vi "Get Cam Focus.vi"() -> ()   [LabVIEW 2015]
uses:
  <vilib>/Utility/file.llb/Read Delimited Spreadsheet (string).vi
  <vilib>/Utility/file.llb/Write Delimited Spreadsheet (string).vi
  Users/Stephen/Desktop/BETA_GSCS - Copy/Systems/SIcamera_Control/SIcamera_Globals.vi
panel:
  in  "Array":string[][](array[string])
  in  "Save":bool
  in  "Line Number":dbl=1.0
  in  "Open script":bool
  in  "Current Script":string[][](table)
  in  "text file":refnum<file>
  in  "Script Name":string
  out "status":string
  in  "Add to Script Button":bool
  in  "Location of Script File":path=path "C:/GSCS Scripting/Scripts"
  in  "cluster":T1={"Path to Configuration File"=path "", "SI camera info"={"Exp time"=0.0, "Number of Exp"=0.0, "Exp type tab"=enum."Object", "CCD ROI Mode"=10, "File name base"="", "Camera Color"="Red", "Notes"="", "Observer Name"="", "object name"="", "CCD Readout Speed"=5, "Hg(Ar)"=FALSE, "Cu"=FALSE, "Ne"=FALSE, "Ar"=FALSE, "Quartz"=FALSE, "Fe"=FALSE, "Bulb"=FALSE, "Quartz Percent"=0.0, "Cam Focus"=0.0}} {"SI camera info"."CCD Readout Speed" items=["750 kHz, ATTN 0", "750 kHz, ATTN 2", "344 kHz, ATTN 0", "344 kHz, ATTN 3", "100 kHz, ATTN 2", "100 kHz, ATTN 3"]; "SI camera info"."CCD ROI Mode" items=["Imaging, 1x1  "=0, "Imaging, 2x2"=1, "Imaging, 3x3"=2, "Spectroscopic, 1x1"=3, "Spectroscopic, 2x2"=4, "Spectroscopic, 3x3"=5, "MOS, 1x1"=11, "MOS, 2x2"=12, "MOS, 3x3"=13, "Slicer"=6, "Spectroscopic, ZZ Ceti"=14, "Slit Imaging/Alignment"=7, "MOS Imaging/Alignment"=10, "Set user-defined ROI..."=21, "Custom Mode"=9]}
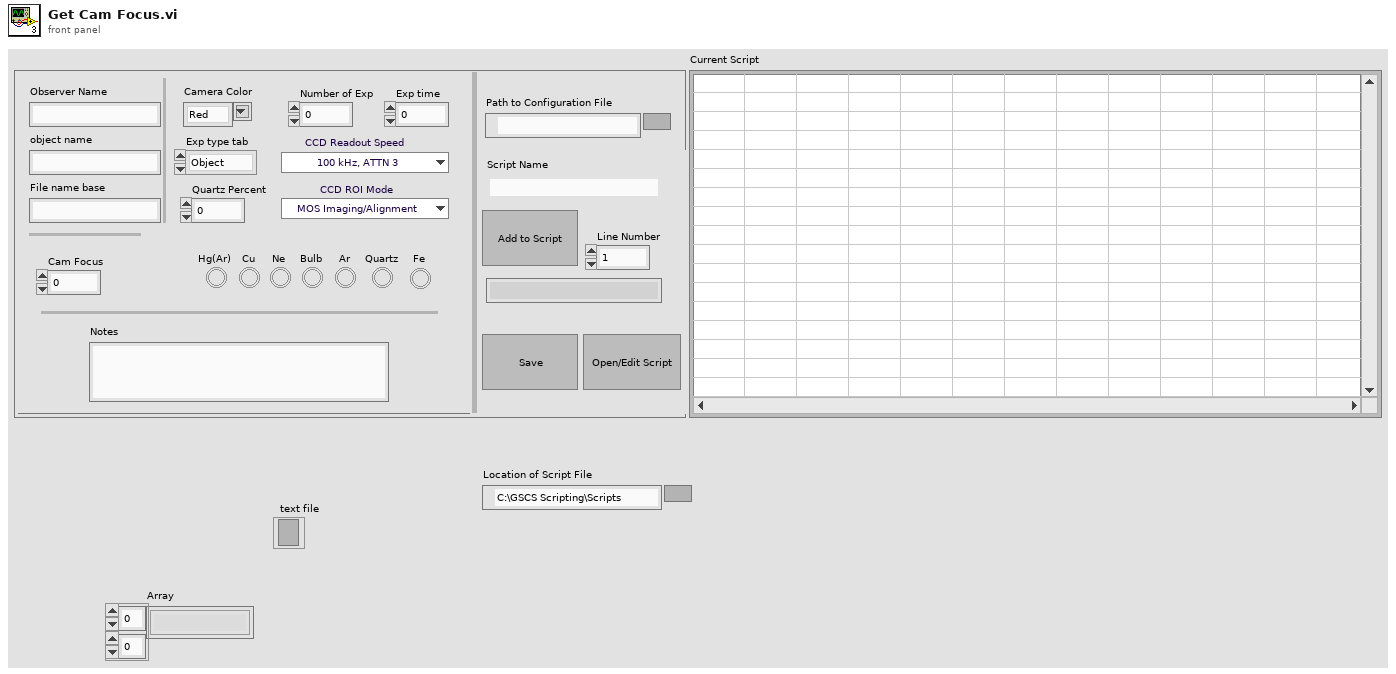
[diagram p1: front panel]
types:
  T1 = cluster{"Path to Configuration File":path, "SI camera info":cluster{"Exp time":dbl, "Number of Exp":dbl, "Exp type tab":enum16{"Object", "Flat", "Comp", "Dark", "Zero"}, "CCD ROI Mode":u16, "File name base":string, "Camera Color":string, "Notes":string, "Observer Name":string, "object name":string, "CCD Readout Speed":u8, "Hg(Ar)":bool, "Cu":bool, "Ne":bool, "Ar":bool, "Quartz":bool, "Fe":bool, "Bulb":bool, "Quartz Percent":dbl, "Cam Focus":dbl}}
  T2 = cluster{"Serial Origin":i32, "Serial Length":i32, "Serial Binning":i32, "Parallel Origin":i32, "Parallel Length":i32, "Parallel Binning":i32}
  T3 = typedef "LVPoint32TypeDef.ctl" = cluster{"Horizontal":i32, "Vertical":i32}
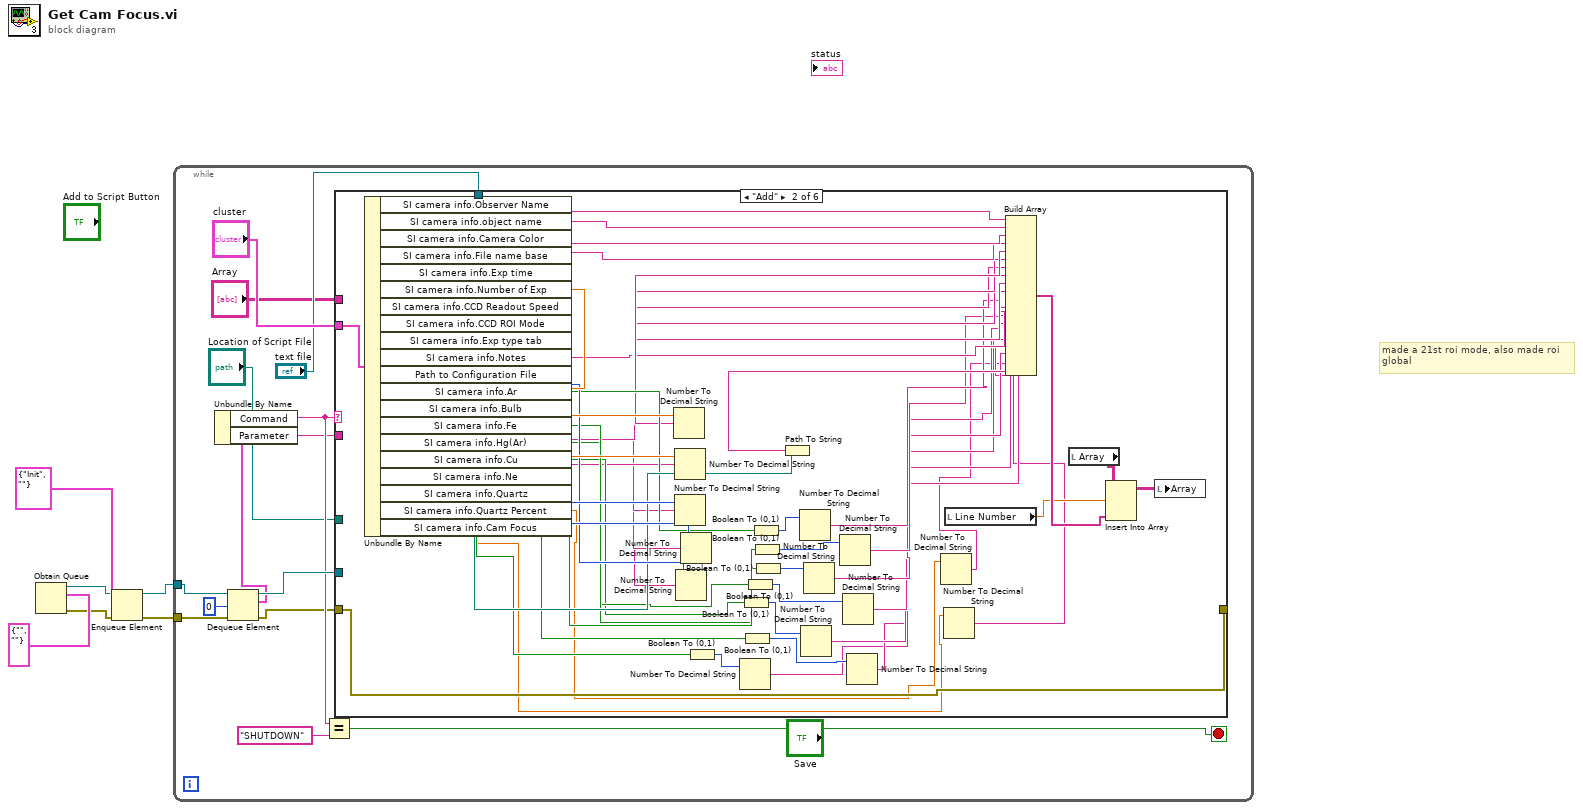
[diagram p0: block diagram]
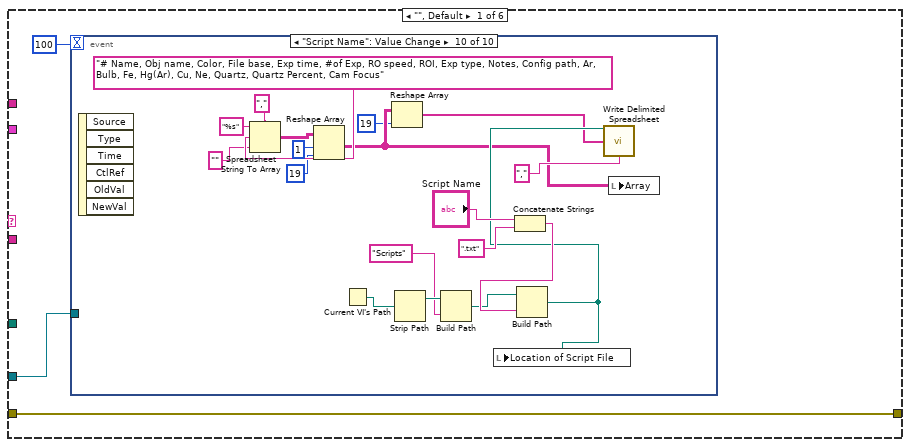
[diagram p2: hidden frame]
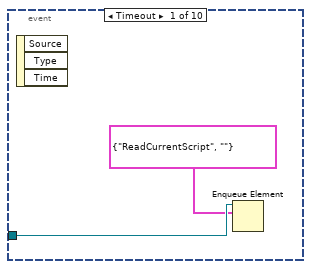
[diagram p3: hidden frame]
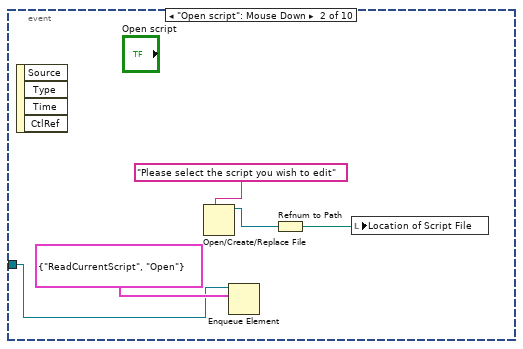
[diagram p4: hidden frame]
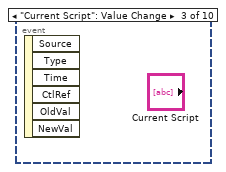
[diagram p5: hidden frame]
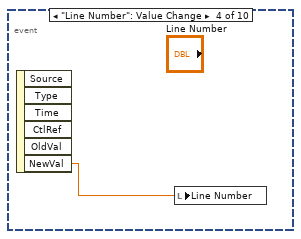
[diagram p6: hidden frame]
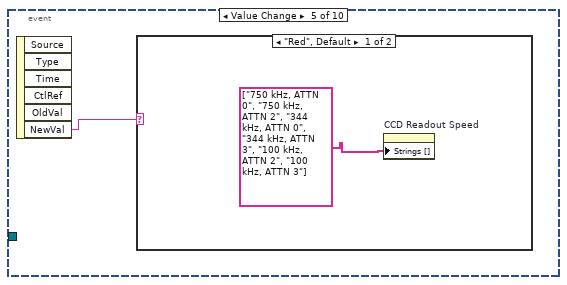
[diagram p7: hidden frame]
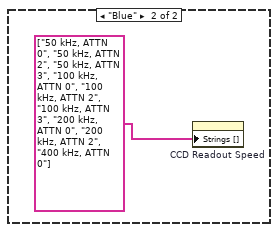
[diagram p8: hidden frame]
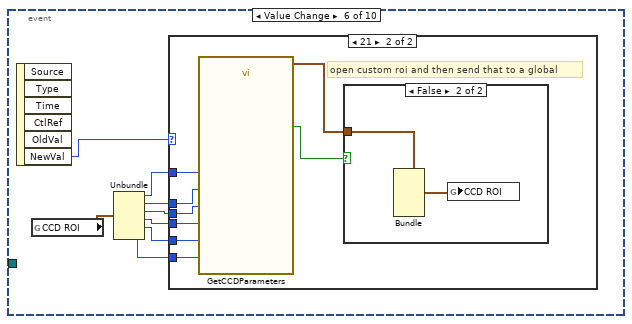
[diagram p9: hidden frame]
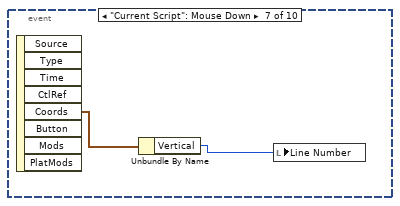
[diagram p12: hidden frame]
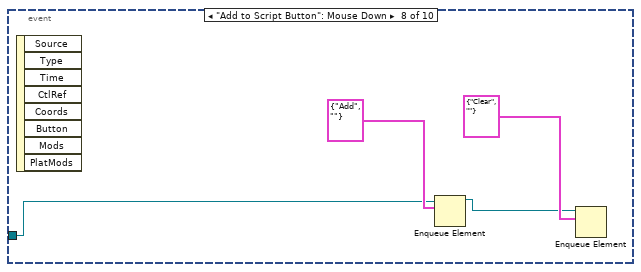
[diagram p13: hidden frame]
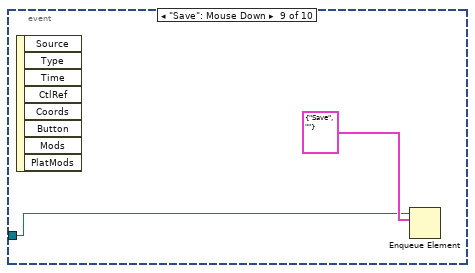
[diagram p14: hidden frame]
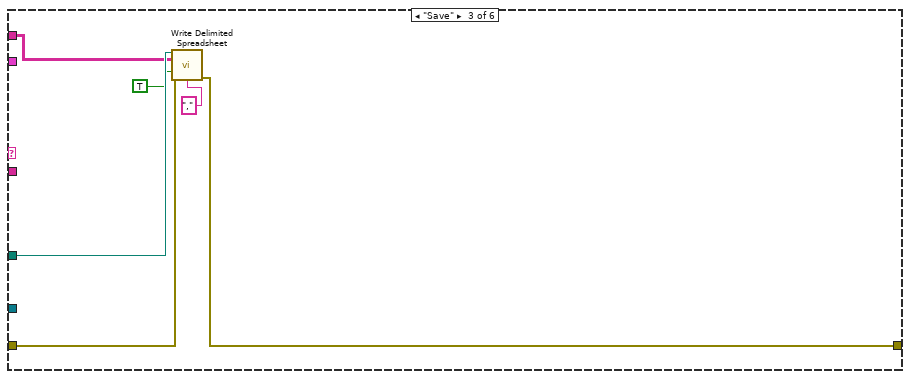
[diagram p15: hidden frame]
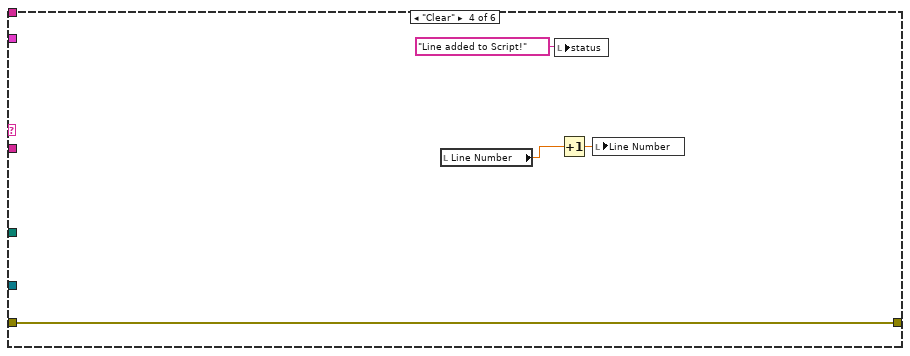
[diagram p16: hidden frame]
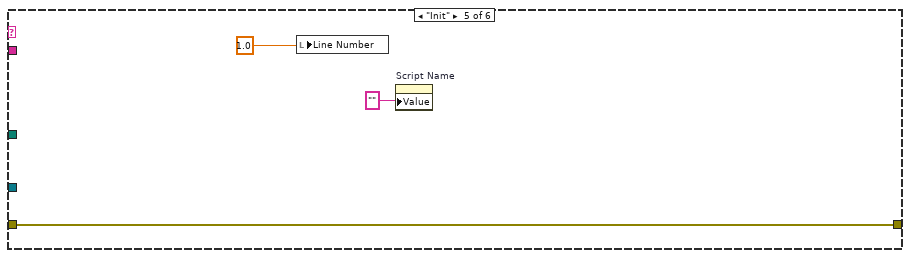
[diagram p17: hidden frame]
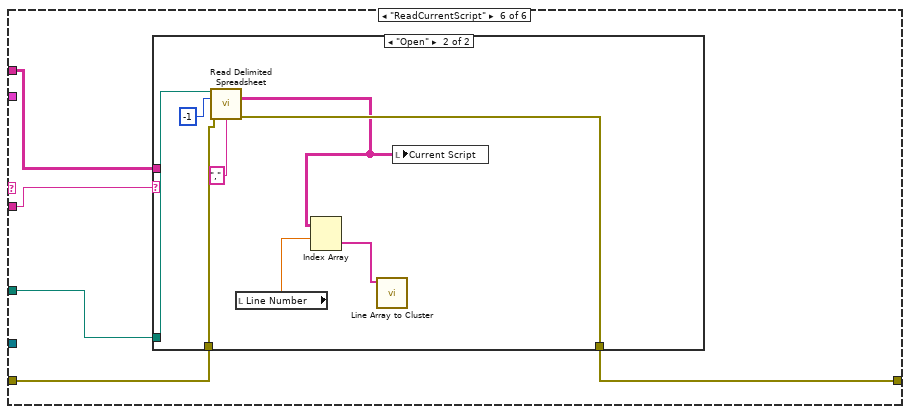
[diagram p18: hidden frame]
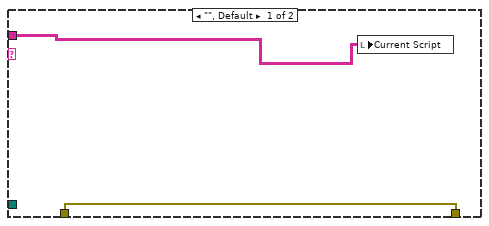
[diagram p19: hidden frame]
diagram:
  # "made a 21st roi mode, also made roi\nglobal"
  n1 = Obtain Queue(element data type=cluster{"\nCommand":string, "Parameter":string} {"\nCommand"="", "Parameter"=""}) -> (queue out=w4:refnum<queue>, error out=w2:errorcluster)  [unwired: 4 in, 1 out]
  n2 = Enqueue Element(queue=w4, element=cluster{string, string} {"Init", ""}, error in (no error)=w2) -> (queue out=w3:refnum<queue>, error out=w1:errorcluster)  [unwired: 1 in, 1 out]
  n3 = while {
    tunnel: w3 -> [w12]
    tunnel: w1 -> [w11]
    stop <- w16 stop-if-true
    n4 = Dequeue Element(queue=w12, timeout in ms (-1)=0, error in (no error)=w11) -> (queue out=w20:refnum<queue>, element=w19:cluster{"\nCommand":string, "Parameter":string}, error out=w10:errorcluster)  [unwired: 1 out]
    n5 = Unbundle By Name(w19) -> ("Command"=w17:string, "Parameter"=w15:string)
    n6 = Equal?(x=w17, y="SHUTDOWN") -> (x = y?=w16:bool)
    n7 = case shown="\"Add\"" w17 {
      tunnel: w20 -> [w23 _ _ _ _ _]
      tunnel: w15 -> [_ _ _ _ _ w142]
      tunnel: "cluster" -> [_ w106 _ _ _ _]
      tunnel: "Location of Script File" -> [_ _ w133 _ _ w145]
      tunnel: w10 -> [w22 w121 w131 w137 w140 w144]
      tunnel: [w22 w121 w130 w137 w140 w143] -> _
      tunnel: "text file" -> [_ _ _ _ _ _]
      tunnel: "Array" -> [_ _ w128 _ _ w141]
      frame "", Default {
        n8 = event shown="[9] \"Script Name\": Value Change" {
          selector: _ -> [_ _ _ _ _ _ _ _ _ _]
          dyn-events: _ -> [_ _ _ _ _ _ _ _ _ _]
          timeout: 100 -> [_ _ _ _ _ _ _ _ _ _]
          tunnel: w23 -> [w25 w26 _ _ _ _ _ w57 w59 _]
          event Timeout {
            n9 = event-data() -> ()  [unwired: 1 in, 3 out]
            n10 = Enqueue Element(queue=w25, element=cluster{string, string} {"ReadCurrentScript", ""}) -> ()  [unwired: 2 in, 3 out]
          }
          event "Open script": Mouse Down {
            n11 = event-data() -> ()  [unwired: 1 in, 4 out]
            n12 = Open/Create/Replace File(prompt="Please select the script you wish to edit") -> (refnum out=w29:refnum<file>)  [unwired: 5 in, 2 out]
            n13 = Enqueue Element(queue=w26, element=cluster{string, string} {"ReadCurrentScript", "Open"}) -> ()  [unwired: 2 in, 3 out]
            n14 = Refnum to Path(1:w29) -> (0:w28:path)
            n15 = local write "Location of Script File"(w28) -> ()
          }
          event "Current Script": Value Change {
            n16 = event-data() -> ()  [unwired: 1 in, 6 out]
          }
          event "Line Number": Value Change {
            n17 = event-data() -> ("NewVal"=w31:dbl)  [unwired: 1 in, 5 out]
            n18 = local write "Line Number"(w31) -> ()
          }
          event "cluster.SI camera info.Camera Color": Value Change {
            n19 = event-data() -> ("NewVal"=w32:string)  [unwired: 1 in, 5 out]
            n20 = case shown="\"Red\", Default" w32 {
              frame "Red", Default {
                n21 = property on="CCD Readout Speed" class="Ring (strict)"("Strings []"=string[] ["750 kHz, ATTN 0", "750 kHz, ATTN 2", "344 kHz, ATTN 0", "344 kHz, ATTN 3", "100 kHz, ATTN 2", "100 kHz, ATTN 3"]) -> ()  [unwired: 2 in, 2 out]
              }
              frame "Blue" {
                n22 = property on="CCD Readout Speed" class="Ring (strict)"("Strings []"=string[] ["50 kHz, ATTN 0", "50 kHz, ATTN 2", "50 kHz, ATTN 3", "100 kHz, ATTN 0", "100 kHz, ATTN 2", "100 kHz, ATTN 3", "200 kHz, ATTN 0", "200 kHz, ATTN 2", "400 kHz, ATTN 0"]) -> ()  [unwired: 2 in, 2 out]
              }
            }
          }
          event "cluster.SI camera info.CCD ROI Mode": Value Change {
            n23 = event-data() -> ("NewVal"=w42:u16)  [unwired: 1 in, 5 out]
            n24 = global read "SIcamera_Globals.vi" "CCD ROI"() -> (w41:cluster{i32, i32, i32, i32, i32, i32})
            n25 = Unbundle(w41) -> (w40:i32, w39:i32, w38:i32, w37:i32, w36:i32, w35:i32)
            n26 = case shown="21" w42 {
              tunnel: w40 -> [_ w50]
              tunnel: w39 -> [_ w49]
              tunnel: w38 -> [_ w48]
              tunnel: w37 -> [_ w47]
              tunnel: w36 -> [_ w46]
              tunnel: w35 -> [_ w45]
              frame 0, Default {
              }
              frame 21 {
                # "open custom roi and then send that to a global"
                n27 = call "GetCCDParameters.vi"("Serial Origin"=w45, "Parallel Origin"=w48, "Serial Length"=w46, "Parallel Length"=w49, "Serial Binning"=w47, "Parallel Binning"=w50) -> ("Cancelled?"=w44:bool, "CCD Format Parameters"=w43:T2)  [unwired: 10 in, 2 out]
                n28 = case shown="False" w44 {
                  tunnel: w43 -> [_ w52]
                  frame True {
                  }
                  frame False {
                    n29 = Bundle(cluster=w52) -> (w51:T2)  [unwired: 6 in]
                    n30 = global write "SIcamera_Globals.vi" "CCD ROI"(w51) -> ()
                  }
                }
              }
            }
          }
          event "Current Script": Mouse Down {
            n31 = event-data() -> ("Coords"=w54:T3)  [unwired: 1 in, 7 out]
            n32 = Unbundle By Name(w54) -> ("Vertical"=w53:i32)
            n33 = local write "Line Number"(w53) -> ()
          }
          event "Add to Script Button": Mouse Down {
            n34 = event-data() -> ()  [unwired: 1 in, 8 out]
            n35 = Enqueue Element(queue=w57, element=cluster{string, string} {"Add", ""}) -> (queue out=w55:refnum<queue>)  [unwired: 2 in, 2 out]
            n36 = Enqueue Element(queue=w55, element=cluster{string, string} {"Clear", ""}) -> ()  [unwired: 2 in, 3 out]
          }
          event "Save": Mouse Down {
            n37 = event-data() -> ()  [unwired: 1 in, 8 out]
            n38 = Enqueue Element(queue=w59, element=cluster{string, string} {"Save", ""}) -> ()  [unwired: 2 in, 3 out]
          }
          event "Script Name": Value Change {
            n39 = event-data() -> ()  [unwired: 1 in, 6 out]
            n40 = Spreadsheet String To Array(delimiter (Tab)=",", format string="%s", spreadsheet string="# Name, Obj name, Color, File base, Exp time, #of Exp, RO speed, ROI, Exp type, Notes, Config path, Ar, Bulb, Fe, Hg(Ar), Cu, Ne, Quartz, Quartz Percent, Cam Focus", array type (2D Dbl)="") -> (array=w66:string[][])
            n41 = Reshape Array(w66, 1, 19) -> (w63:string[][])
            n42 = Current VI's Path() -> (path=w79:path)
            n43 = Reshape Array(w63, 19) -> (w61:string[])
            n44 = Strip Path(path=w79) -> (stripped path=w78:path)  [unwired: 1 out]
            n45 = Build Path(base path=w78, name or relative path="Scripts") -> (appended path=w73:path)
            n46 = Concatenate Strings("Script Name", ".txt") -> (w74:string)
            n47 = Build Path(base path=w73, name or relative path=w74) -> (appended path=w72:path)
            n48 = local write "Location of Script File"(w72) -> ()
            n49 = call-poly <vilib>:"Write Delimited Spreadsheet.vi"("file path (dialog if empty)"=w72, "1D data"=w61, "delimiter (\\t)"=",") -> ()  [unwired: 11 in, 2 out]
            n50 = local write "Array"(w63) -> ()
          }
        }
      }
      frame "Add" {
        n51 = Unbundle By Name(w106) -> ("SI camera info.Observer Name"=w105:string, "SI camera info.object name"=w104:string, "SI camera info.Camera Color"=w103:string, "SI camera info.File name base"=w102:string, "SI camera info.Exp time"=w127:dbl, "SI camera info.Number of Exp"=w126:dbl, "SI camera info.CCD Readout Speed"=w125:u8, "SI camera info.CCD ROI Mode"=w124:u16, "SI camera info.Exp type tab"=w123:enum16{"Object", "Flat", "Comp", "Dark", "Zero"}, "SI camera info.Notes"=w96:string, "Path to Configuration File"=w122:path, "SI camera info.Ar"=w120:bool, "SI camera info.Bulb"=w118:bool, "SI camera info.Fe"=w116:bool, "SI camera info.Hg(Ar)"=w114:bool, "SI camera info.Cu"=w112:bool, "SI camera info.Ne"=w110:bool, "SI camera info.Quartz"=w108:bool, "SI camera info.Quartz Percent"=w83:dbl, "SI camera info.Cam Focus"=w82:dbl)
        n52 = Number To Decimal String(number=w127) -> (decimal integer string=w101:string)  [unwired: 1 in]
        n53 = Number To Decimal String(number=w126) -> (decimal integer string=w100:string)  [unwired: 1 in]
        n54 = Number To Decimal String(number=w125) -> (decimal integer string=w99:string)  [unwired: 1 in]
        n55 = Number To Decimal String(number=w123) -> (decimal integer string=w97:string)  [unwired: 1 in]
        n56 = Number To Decimal String(number=w124) -> (decimal integer string=w98:string)  [unwired: 1 in]
        n57 = Boolean To (0,1)(Boolean=w108) -> (0, 1=w107:i16)
        n58 = Number To Decimal String(number=w107) -> (decimal integer string=w88:string)  [unwired: 1 in]
        n59 = Boolean To (0,1)(Boolean=w112) -> (0, 1=w111:i16)
        n60 = Boolean To (0,1)(Boolean=w110) -> (0, 1=w109:i16)
        n61 = Boolean To (0,1)(Boolean=w114) -> (0, 1=w113:i16)
        n62 = Boolean To (0,1)(Boolean=w120) -> (0, 1=w119:i16)
        n63 = Boolean To (0,1)(Boolean=w118) -> (0, 1=w117:i16)
        n64 = Boolean To (0,1)(Boolean=w116) -> (0, 1=w115:i16)
        n65 = Path To String(path=w122) -> (string=w95:string)
        n66 = Number To Decimal String(number=w119) -> (decimal integer string=w94:string)  [unwired: 1 in]
        n67 = Number To Decimal String(number=w111) -> (decimal integer string=w90:string)  [unwired: 1 in]
        n68 = Number To Decimal String(number=w115) -> (decimal integer string=w92:string)  [unwired: 1 in]
        n69 = Number To Decimal String(number=w117) -> (decimal integer string=w93:string)  [unwired: 1 in]
        n70 = Number To Decimal String(number=w113) -> (decimal integer string=w91:string)  [unwired: 1 in]
        n71 = Number To Decimal String(number=w109) -> (decimal integer string=w89:string)  [unwired: 1 in]
        n72 = Number To Decimal String(number=w83) -> (decimal integer string=w81:string)  [unwired: 1 in]
        n73 = Number To Decimal String(number=w82) -> (decimal integer string=w80:string)  [unwired: 1 in]
        n74 = local read "Line Number"() -> (w85:dbl)
        n75 = Build Array(w105, w104, w103, w102, w101, w100, w99, w98, w97, w96, w95, w94, w93, w92, w91, w90, w89, w88, w81, w80) -> (w87:string[])
        n76 = local read "Array"() -> (w84:string[][])
        n77 = Insert Into Array(array=w84, index (row)=w85, new element=w87) -> (w86:string[][])  [unwired: 1 in]
        n78 = local write "Array"(w86) -> ()
      }
      frame "Save" {
        n79 = call-poly <vilib>:"Write Delimited Spreadsheet.vi"("file path (dialog if empty)"=w133, "2D data"=w128, "append to file? (F)"=TRUE, "error in (no error)"=w131, "delimiter (\\t)"=",") -> ("error out"=w130:errorcluster)  [unwired: 9 in, 1 out]
      }
      frame "Clear" {
        n80 = local read "Line Number"() -> (w134:dbl)
        n81 = local write "status"("Line added to Script!") -> ()
        n82 = Increment(x=w134) -> (x+1=w135:dbl)
        n83 = local write "Line Number"(w135) -> ()
      }
      frame "Init" {
        n84 = local write "Line Number"(1.0) -> ()
        n85 = property on="Script Name" class="Str"("Value"="") -> ()  [unwired: 2 in, 2 out]
      }
      frame "ReadCurrentScript" {
        n86 = case shown="\"Open\"" w142 {
          tunnel: w145 -> [_ w153]
          tunnel: w144 -> [w147 w152]
          tunnel: [w147 w151] -> w143
          tunnel: w141 -> [w146 _]
          frame "", Default {
            n87 = local write "Current Script"(w146) -> ()
          }
          frame "Open" {
            n88 = call-poly <vilib>:"Read Delimited Spreadsheet.vi"("file path (dialog if empty)"=w153, "number of rows (all:-1)"=-1, "error in (no error)"=w152, "delimiter (\\t)"=",") -> ("all rows"=w150:string[][], "error out"=w151:errorcluster)  [unwired: 6 in, 4 out]
            n89 = local read "Line Number"() -> (w149:dbl)
            n90 = Index Array(array=w150, index (row)=w149) -> (element=w148:string[])  [unwired: 1 in]
            n91 = call "Line Array to Cluster.vi"("Array"=w148) -> ()  [unwired: 10 in, 1 out]
            n92 = local write "Current Script"(w150) -> ()
          }
        }
      }
    }
  }
